vi "Skip scheduled cell.vi"(8 "error in (no error)":errorcluster, 11 "Monkey in":refnum<class "Monkey.lvclass">) -> (0 "error out":errorcluster, 2 "Skipped Run":refnum<class "Run Instance.lvclass">, 3 "Monkey out":refnum<class "Monkey.lvclass">)   [LabVIEW 2020, in "Monkey.lvlib" / "Monkey.lvclass"]
doc: "Moves entire schedule cell to the skipped list"
uses:
  Monkey.lvclass
  Run Utilities/Run Instance/Run Instance.lvclass
  Run Utilities/Run Block/Run Block.lvclass
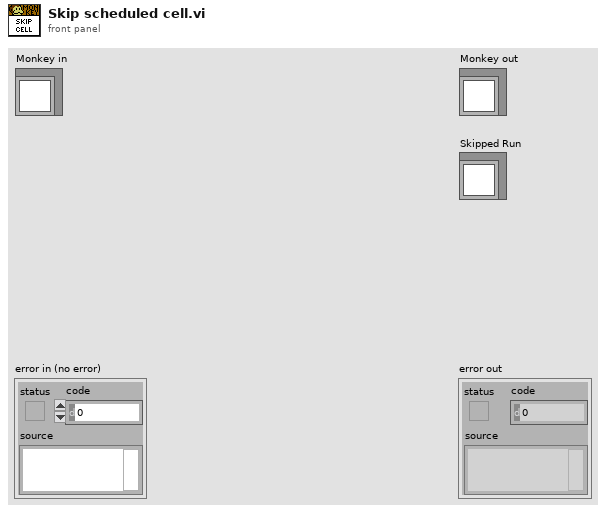
[diagram p1: front panel]
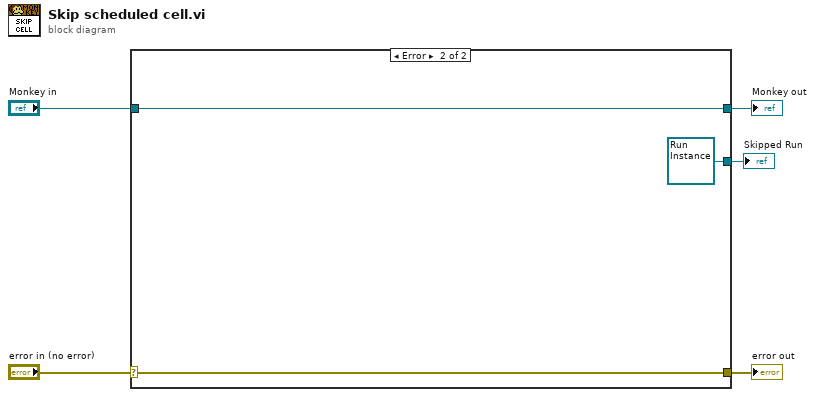
[diagram p0: block diagram]
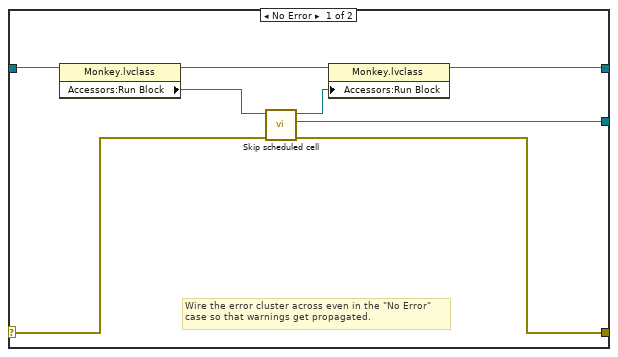
[diagram p2: hidden frame]
diagram:
  n1 = case shown="Error" "error in (no error)" {
    selector: "error in (no error)" -> [w9 w16]
    tunnel: [w10 w16] -> w4
    tunnel: [w12 w15] -> w2
    tunnel: "Monkey in" -> [w13 w15]
    tunnel: [w6 refnum<class "Run Instance.lvclass"> refnum ("Skipped Run")] -> w1
    frame No Error {
      # "Wire the error cluster across even in the \"No Error\"\ncase so that warnings get propagated."
      n2 = property class="Monkey.lvclass"(reference=w13) -> (reference out=w7:refnum<class "Monkey.lvclass">, "Accessors:Run Block"=w8:refnum<class "Run Block.lvclass">)  [unwired: 1 in, 1 out]
      n3 = call-dynamic "Skip scheduled cell.vi"("error in (no error)"=w9, "Run Block in"=w8) -> ("error out"=w10:errorcluster, "Skipped Run"=w6:refnum<class "Run Instance.lvclass">, "Run Block out"=w11:refnum<class "Run Block.lvclass">)  [unwired: 7 in]
      n4 = property class="Monkey.lvclass"(reference=w7, "Accessors:Run Block"=w11) -> (reference out=w12:refnum<class "Monkey.lvclass">)  [unwired: 1 in, 1 out]
    }
    frame Error {
    }
  }
  "error out" <- w4
  "Monkey out" <- w2
  "Skipped Run" <- w1
